vi "M Smart Grid.vi"(11 "EV3 in":T1) -> (3 "EV3 out":T1)   [LabVIEW 2016]
uses:
  <vilib>/NXT/Subs/LVHSConnector.ctl
  <vilib>/NXT/LegoClasses/BrickReference/BrickReference.lvclass
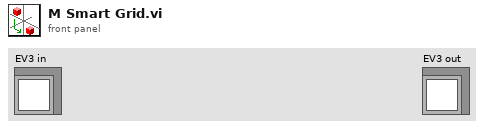
[diagram p1: front panel]
types:
  T1 = typedef "LVHSConnector.ctl" = refnum<class "BrickReference.lvclass">
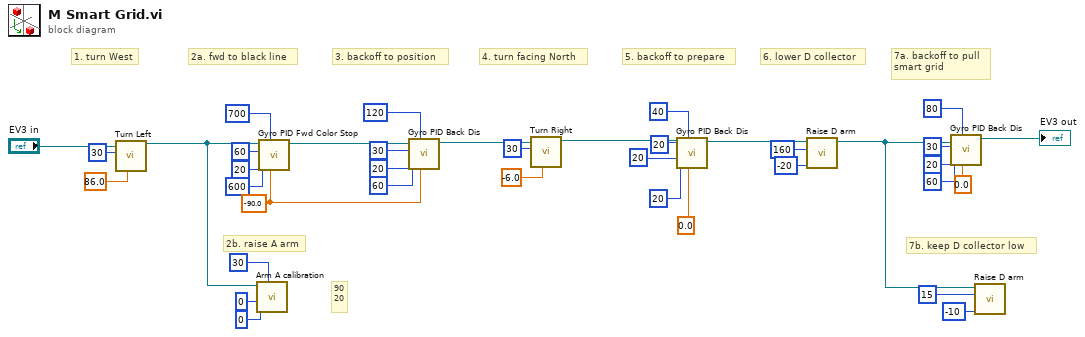
[diagram p0: block diagram]
diagram:
  w26 = sgl -90.0 ("Target angle")
  # "90\n20"
  # "7b. keep D collector low"
  # "7a. backoff to pull\nsmart grid"
  # "6. lower D collector"
  # "5. backoff to prepare"
  # "4. turn facing North"
  # "3. backoff to position"
  # "2b. raise A arm"
  # "2a. fwd to black line"
  # "1. turn West"
  n1 = call "Turn Left.vi"("Turning angle"=sgl 86.0, "Motor B (right)"=i8 30, "EV3 in"="EV3 in") -> ("EV3 out"=w32:T1)  [unwired: 8 in]
  n2 = call "Arm A calibration.vi"("Cali. Power"=i8 30, "Down Power"=i8 0, "Rotation"=0, "NXT/EV3"=w32) -> ()  [unwired: 7 in, 1 out]
  n3 = call "Gyro PID Fwd Color Stop.vi"("Target angle"=w26, "Threshold to Color"=700, "Threshold to slow"=600, "Min. speed"=20, "Max. speed"=60, "EV3 in"=w32) -> ("EV3 out"=w31:T1)  [unwired: 5 in]
  n4 = call "Gyro PID Back Dis.vi"("Target angle"=w26, "Threshold to stop"=120, "Threshold to slow"=60, "Min. speed"=20, "Max. speed"=30, "EV3 in"=w31) -> ("EV3 out"=w25:T1)  [unwired: 5 in]
  n5 = call "Turn Right.vi"("Turning angle"=sgl -6.0, "Motor B (right)"=i8 30, "EV3 in"=w25) -> ("EV3 out"=w22:T1)  [unwired: 8 in]
  n6 = call "Gyro PID Back Dis.vi"("Target angle"=sgl 0.0, "Threshold to stop"=40, "Threshold to slow"=20, "Min. speed"=20, "Max. speed"=20, "EV3 in"=w22) -> ("EV3 out"=w16:T1)  [unwired: 5 in]
  n7 = call "Raise D arm.vi"("Power"=i8 -20, "Rotation"=160, "EV3 in"=w16) -> ("EV3 out"=w8:T1)  [unwired: 8 in]
  n8 = call "Gyro PID Back Dis.vi"("Target angle"=sgl 0.0, "Threshold to stop"=80, "Threshold to slow"=60, "Min. speed"=20, "Max. speed"=30, "EV3 in"=w8) -> ("EV3 out"=→"EV3 out":T1)  [unwired: 5 in]
  n9 = call "Raise D arm.vi"("Power"=i8 -10, "Rotation"=15, "EV3 in"=w8) -> ()  [unwired: 8 in, 1 out]
